vi "Close.vi"(8 "error in":errorcluster, 11 "Cell View Back Color Alternate in":refnum<class "Cell View Back Color Alternate.lvclass">) -> (0 "error out":errorcluster, 3 "Cell View Back Color Alternate out":refnum<class "Cell View Back Color Alternate.lvclass">)   [LabVIEW 2024, in "PDO Grid.lvlib" / "Cell View Back Color Alternate.lvclass"]
uses:
  Cell View Back Color Alternate.lvclass
  Sourcegrid-LabVIEW/source/Views/ViewBase/Cell View.lvclass
  Cell View Back Color Alternate.lvclass/Cell View Back Color Alternate.ctl
  Sourcegrid-LabVIEW/source/Color/Color.lvclass
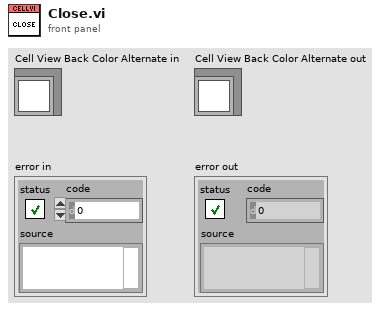
[diagram p1: front panel]
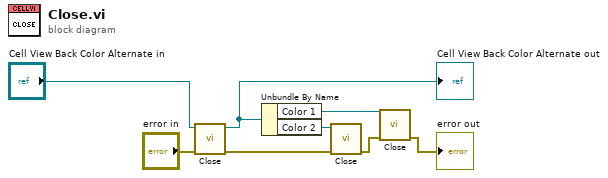
[diagram p0: block diagram]
diagram:
  n1 = call-parent "Close.vi"("error in"="error in", "Cell View in"="Cell View Back Color Alternate in") -> ("error out"=w2:errorcluster, "Cell View out"=w6:refnum<class "Cell View Back Color Alternate.lvclass">)  [unwired: 8 in]
  "Cell View Back Color Alternate out" <- w6
  n2 = Unbundle By Name(w6) -> ("Color 1"=w3:refnum<class "Color.lvclass">, "Color 2"=w5:refnum<class "Color.lvclass">)
  n3 = call-dynamic "Close.vi"("error in"=w2, "Color in"=w5) -> ("error out"=w4:errorcluster)  [unwired: 8 in, 1 out]
  n4 = call-dynamic "Close.vi"("error in"=w4, "Color in"=w3) -> ("error out"=→"error out":errorcluster)  [unwired: 8 in, 1 out]
